vi "Problem 7 - 10001st prime.vi"(8 "error in (no error)":errorcluster) -> (0 "error out":errorcluster, 2 "Execution time (ms)":u32, 3 "Answer":i32)   [LabVIEW 2021, in "Project Euler.lvlib"]
uses:
  Project Euler.lvlib
  Utilities/Named Timers/Named Timers.lvlib
  Utilities/Numeric Utilities/Numeric Utilities.lvlib
panel:
  out "Number of primes":i32
  # "Development\ncontrols/indicators useful for development and testing, but which are not outputs of the VI"
  # "Input\nInputs to the VI"
  # "Output\nOutputs of the VI"
  # "Description\n\nBlank VI with error handling case. \n\nSummarize the use of this VI in this space."
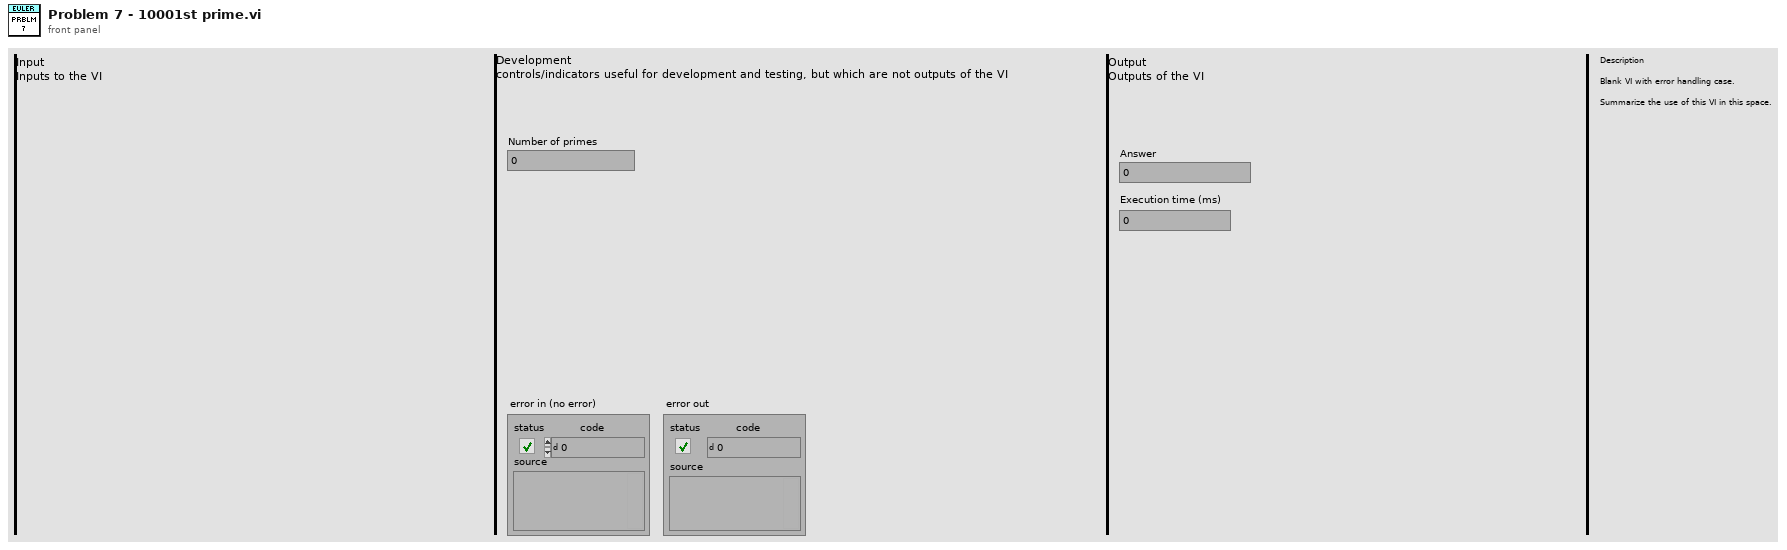
[diagram p1: front panel]
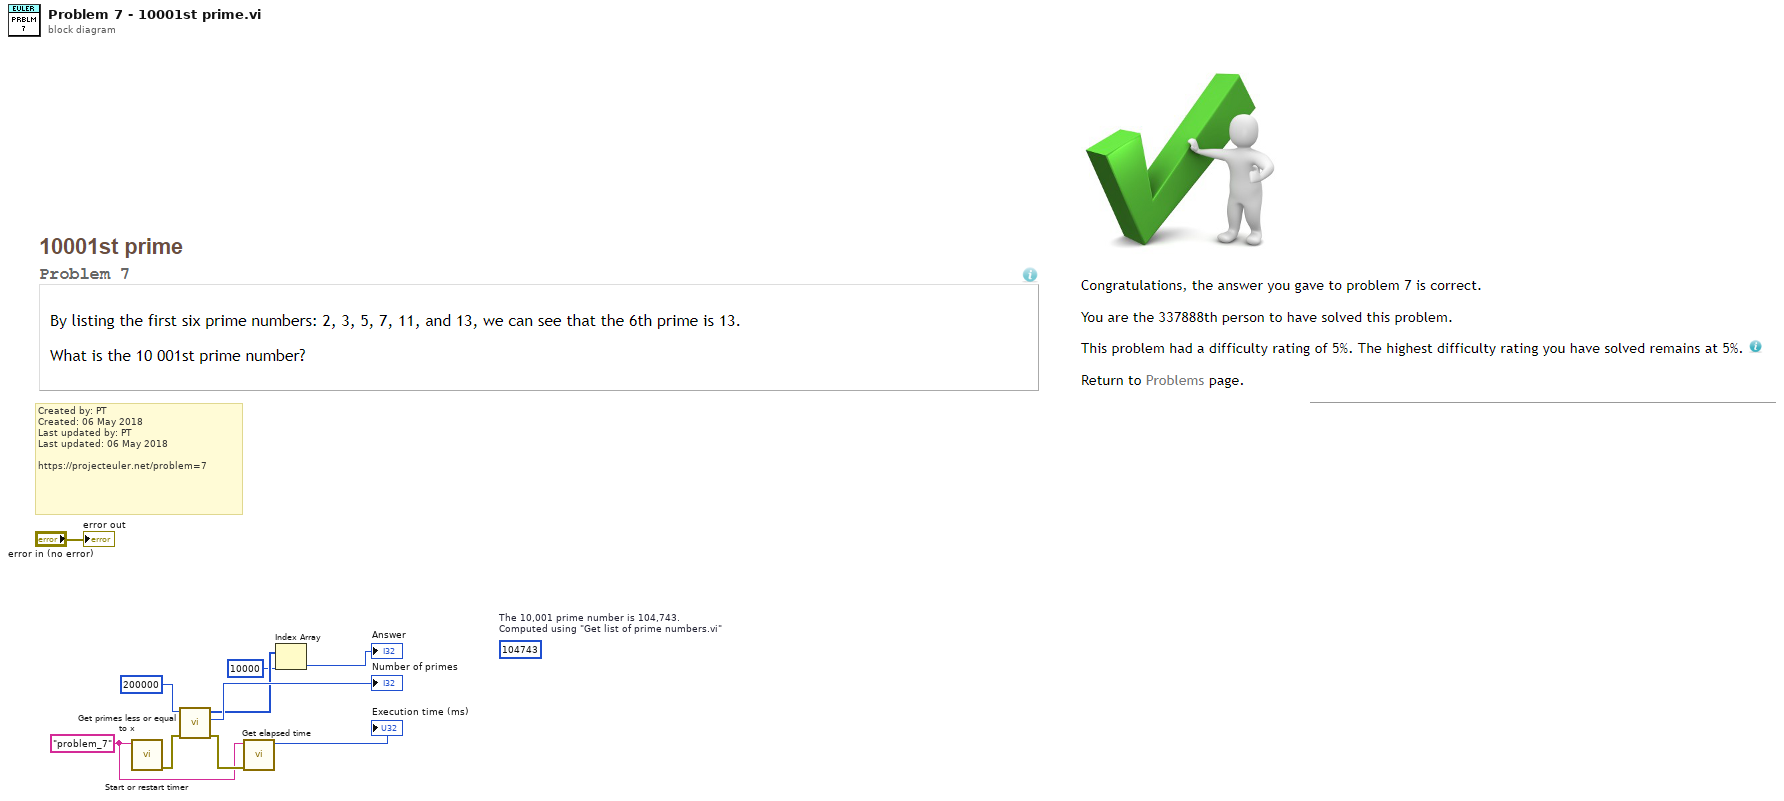
[diagram p0: block diagram]
diagram:
  w1 = "problem_7" ("Timer name")
  (unwired) 104743  # The 10,001 prime number is 104,743. Computed using "Get list of prime numbers.vi"
  # "Created by: PT\nCreated: 06 May 2018\nLast updated by: PT\nLast updated: 06 May 2018\n\nhttps://projecteuler.net/problem=7"
  n1 = call "Start or restart timer.vi"("Timer name"=w1) -> ("error out"=w3:errorcluster)  [unwired: 10 in]
  n2 = call "Get primes less or equal to x.vi"("error in (no error)"=w3, "x = end"=200000) -> ("error out"=w2:errorcluster, "Number of primes"=→"Number of primes":i32, "Primes"=w6:i32[])  [unwired: 7 in]
  n3 = call "Get elapsed time.vi"("error in (no error)"=w2, "Timer name"=w1) -> ("Elapsed time (ms)"=→"Execution time (ms)":u32)  [unwired: 6 in, 3 out]
  n4 = Index Array(array=w6, index=10000) -> (element=→"Answer":i32)
  "error out" <- "error in (no error)"
